vi "Get-state-string.vi"(11 "States":T1) -> (3 "State string":string)   [LabVIEW 2013, in "HardwareCharacterization.lvlib" / "HC-UI.lvclass"]
uses:
  HC-UI.lvclass
  Main/Main-actions.ctl
  Main/HC-Main.lvclass
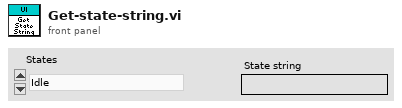
[diagram p1: front panel]
types:
  T1 = typedef "HardwareCharacterization.lvlib/HC-Main.lvclass/Main-actions.ctl" = enum16{"Idle", "Initialize", "Load configuration", "Save configuration", "Load file", "Edit settings", "View scan file", "View raw path", "Edit measurement settings", "Activate", "Start", "Stop", "Refresh display", "Exit"}
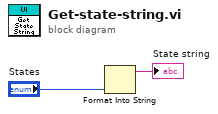
[diagram p0: block diagram]
diagram:
  n1 = Format Into String("States") -> (resulting string=→"State string":string)  [unwired: 3 in, 1 out]
